vi "Oscilloscope.vi"() -> ()   [LabVIEW 2020]
uses:
  Queues4Osc.ctl
  <instrlib>/Tektronix TDS 200 1000 2000 Series/Public/Configure/Configure Trigger (Edge).vi
  <instrlib>/Tektronix TDS 200 1000 2000 Series/Tektronix TDS 200 1000 2000 Series.lvlib
panel:
  in  "VISA resource name":refnum<visa-resource-name>
  in  "stop":bool
  in  "Auto Set":bool
  in  "Measure Parameters":T1 {"Measurement Type" items=["Frequency"=0, "Period"=2, "Pk-Pk"=4, "Cycle RMS"=5]}
  in  "Trigger Parameters":T2 {"Trigger Level" min=-200.0 max=200.0 scale=-200.0..200.0}
  in  "Horizontal Parameters":T3 {"Horizontal Scale" items=["5ns"=200000000.0, "10ns"=100000000.0, "25ns"=40000000.0, "50ns"=20000000.0, "100ns"=10000000.0, "250ns"=4000000.0, "500ns"=2000000.0, "1us"=1e-06, "2.5us"=3e-06, "5us"=5e-06, "10us"=1e-05, "25us"=2.5e-05, "50us"=5e-05, "100us"=0.0001, "250us"=0.00025, "500us"=0.0005, "1ms"=0.001, "2.5ms"=0.0025, "5ms"=0.005, "10ms"=0.01, "25ms"=0.025, "50ms"=0.05, "100ms"=0.1, "250ms"=0.25, "500ms"=0.5, "1s"=1.0, "2.5s"=2.5, "5s"=5.0, "10s"=10.0, "25s"=25.0, "50s"=50.0]; "Horizontal Position" min=-1.0 max=1.0 scale=-1.0..1.0}
  in  "Vertical Parameters":T4 {"Ch2 Vertical Scale" items=["20mV"=500.0, "50mV"=200.0, "100mV"=100.0, "200mV"=50.0, "500mV"=20.0, "1V"=10.0, "2V"=5.0, "5V"=2.0, "10V"=1.0, "20V"=0.5, "50V"=0.2]; "Ch1 Vertical Scale" items=["20mV"=500.0, "50mV"=200.0, "100mV"=100.0, "200mV"=50.0, "500mV"=20.0, "1V"=10.0, "2V"=5.0, "5V"=2.0, "10V"=1.0, "20V"=0.5, "50V"=0.2]}
  out "Channel 2":waveform(dbl)(graph)
  out "Channel 1":waveform(dbl)(graph)
  # "Measure Parameters"
  # "Trigger Parameters"
  # "Horizontal Parameters"
  # "Vertical Parameters"
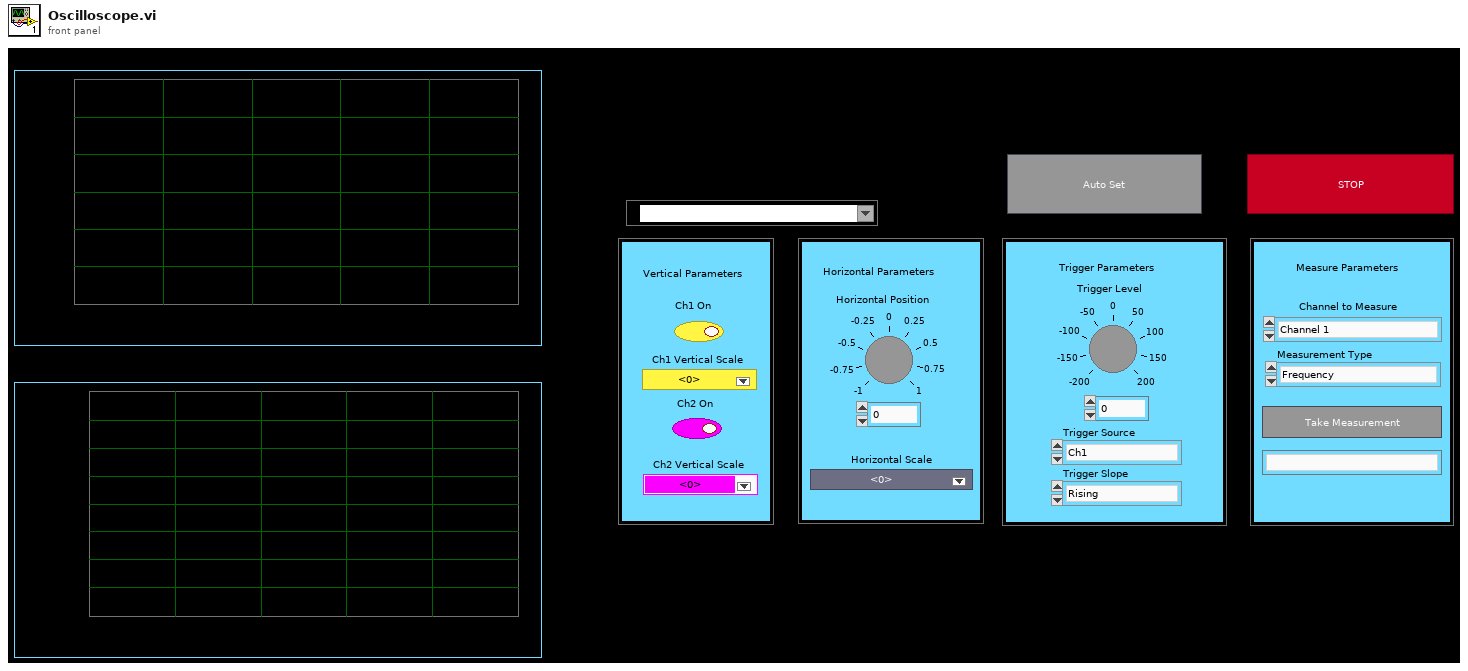
[diagram p1: front panel]
types:
  T1 = cluster{"Channel to Measure":enum16{"Channel 1", "Channel 2"}, "Take Measurement":bool, "String":string, "Measurement Type":u16}
  T2 = cluster{"Trigger Level":dbl, "Trigger Source":enum16{"Ch1", "Ch2"}, "Trigger Slope":enum16{"Rising", "Falling"}}
  T3 = cluster{"Horizontal Position":dbl, "Horizontal Scale":dbl}
  T4 = cluster{"Ch1 On":bool, "Ch2 On":bool, "Ch1 Vertical Scale":dbl, "Ch2 Vertical Scale":dbl}
  T5 = typedef "Queues4Osc.ctl" = enum16{"Initialize", "Idle", "Channels", "Horizontal", "Trigger", "Measure", "Autoset", "Stop"}
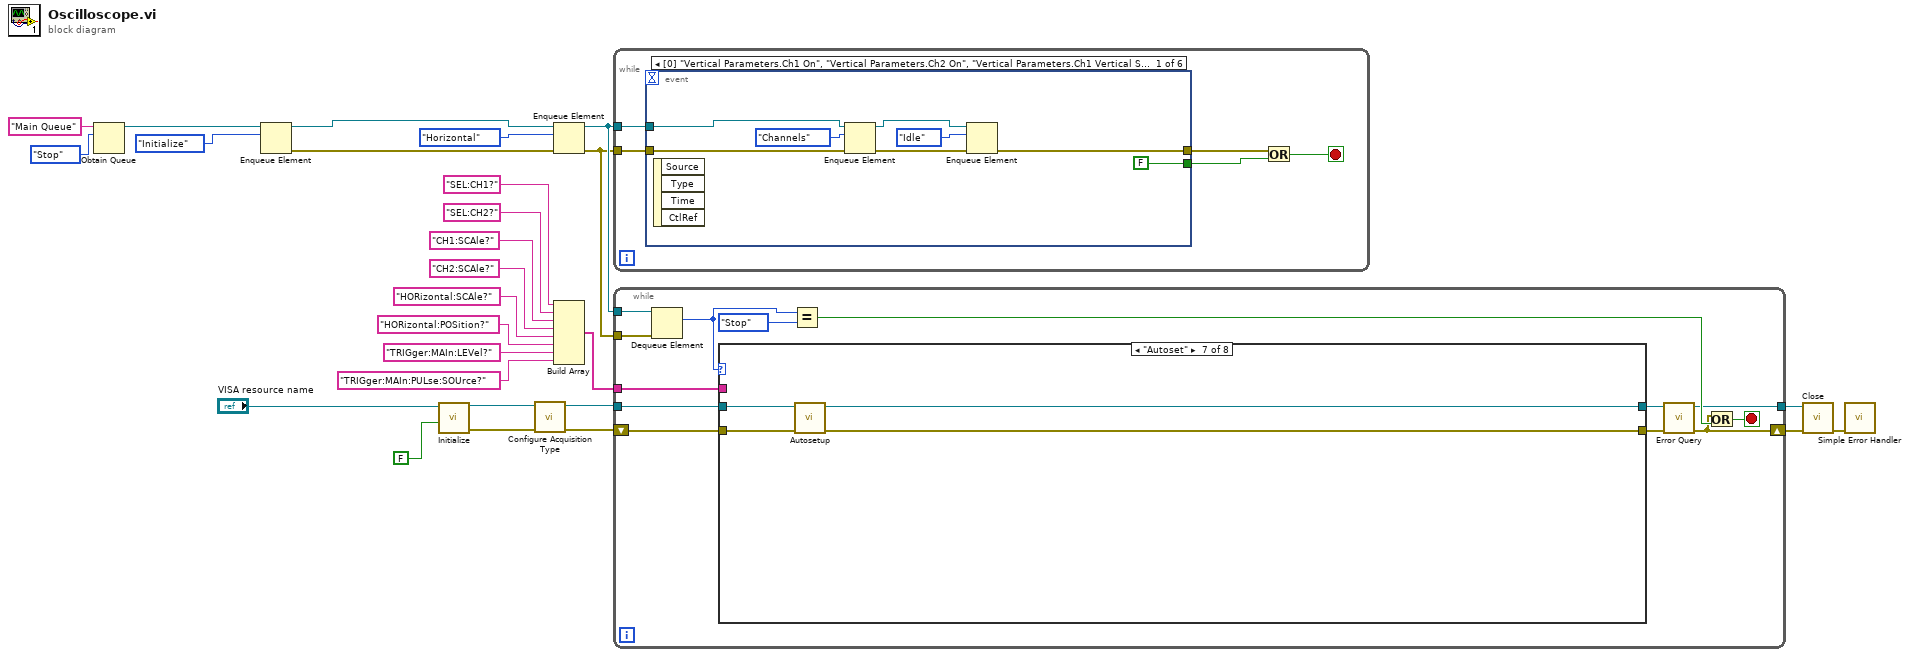
[diagram p0: block diagram]
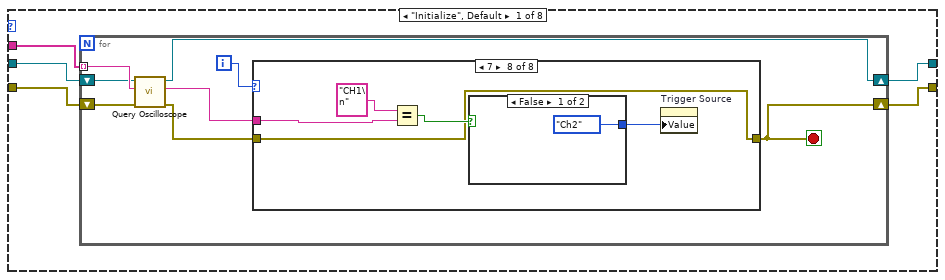
[diagram p2: hidden frame]
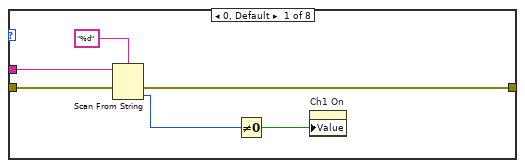
[diagram p3: hidden frame]
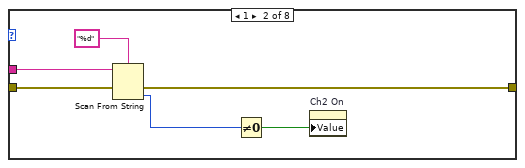
[diagram p4: hidden frame]
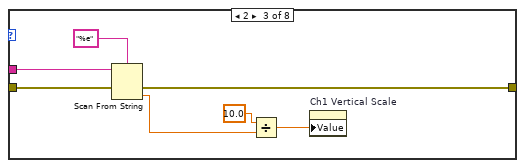
[diagram p5: hidden frame]
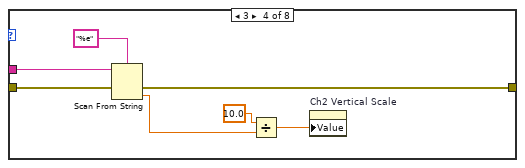
[diagram p6: hidden frame]
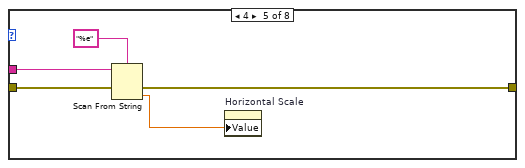
[diagram p7: hidden frame]
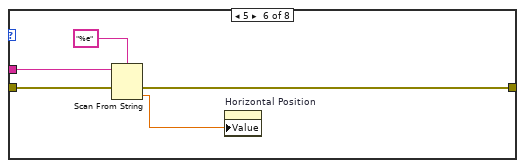
[diagram p8: hidden frame]
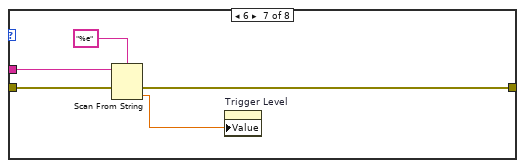
[diagram p9: hidden frame]
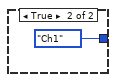
[diagram p10: hidden frame]
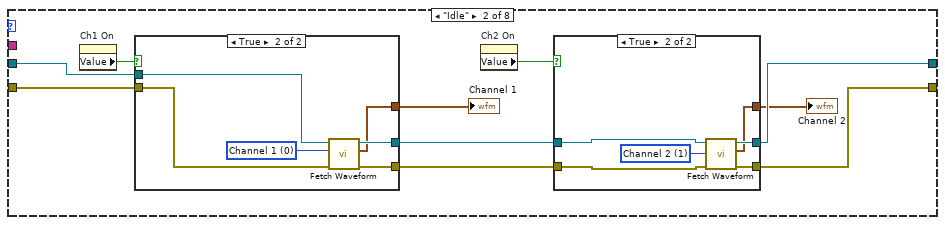
[diagram p11: hidden frame]
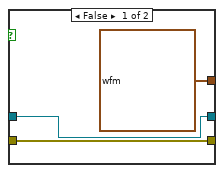
[diagram p12: hidden frame]
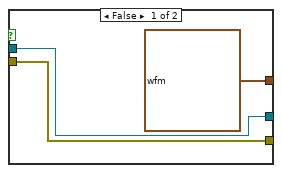
[diagram p13: hidden frame]
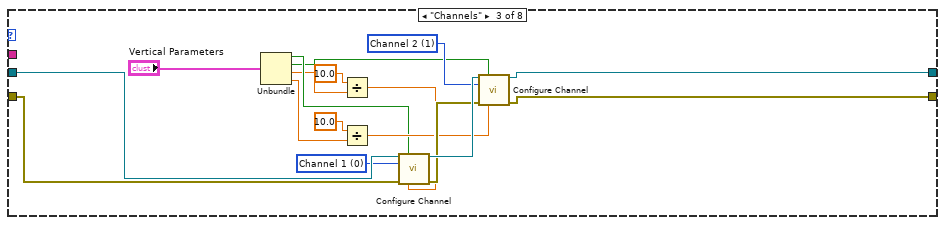
[diagram p14: hidden frame]
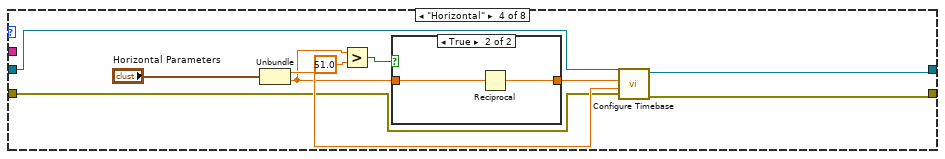
[diagram p15: hidden frame]
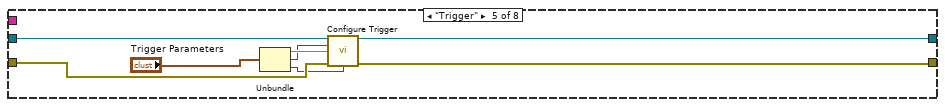
[diagram p17: hidden frame]
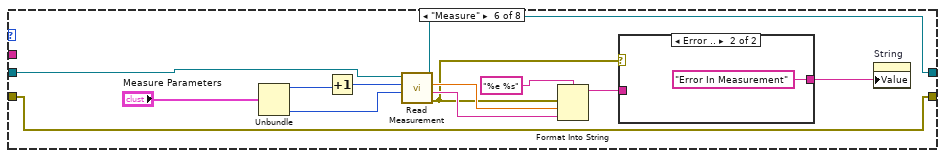
[diagram p18: hidden frame]
diagram:
  n1 = Obtain Queue(name (unnamed)="Main Queue", element data type=Queues4Osc."Stop") -> (queue out=w25:refnum<queue>)  [unwired: 3 in, 2 out]
  n2 = Enqueue Element(queue=w25, element=Queues4Osc."Initialize") -> (queue out=w8:refnum<queue>, error out=w9:errorcluster)  [unwired: 2 in, 1 out]
  n3 = call <instrlib>:"Initialize.vi"("Reset? (T: Yes)"=FALSE, "VISA resource name"="VISA resource name") -> ("error out"=w1:errorcluster, "VISA resource name out"=w2:refnum<visa-resource-name>)  [unwired: 8 in]
  n4 = call <instrlib>:"Configure Acquisition Type.vi"("error in (no error)"=w1, "VISA resource name"=w2) -> ("error out"=w3:errorcluster, "VISA resource name out"=w4:refnum<visa-resource-name>)  [unwired: 8 in]
  n5 = Enqueue Element(queue=w8, element=Queues4Osc."Horizontal", error in (no error)=w9) -> (queue out=w6:refnum<queue>, error out=w5:errorcluster)  [unwired: 1 in, 1 out]
  n6 = Build Array("SEL:CH1?" ("Input Command"), "SEL:CH2?", "CH1:SCAle?", "CH2:SCAle?", "HORizontal:SCAle?", "HORizontal:POSition?", "TRIGger:MAIn:LEVel?", "TRIGger:MAIn:PULse:SOUrce?") -> (w11:string[])
  n7 = while {
    tunnel: w6 -> [w32]
    tunnel: w5 -> [w31]
    stop <- w30 stop-if-true
    n8 = event shown="[0] \"Vertical Parameters.Ch1 On\", \"Vertical Parameters.Ch2 On\", \"Vertical Parameters.Ch1 Vertical Scale\", \"Vertical Parameters.Ch2 Vertical Scale\": Value Change" {
      selector: _ -> [_ _ _ _ _ _]
      dyn-events: _ -> [_ _ _ _ _ _]
      timeout: _ -> [_ _ _ _ _ _]
      tunnel: w32 -> [w40 w44 w52 w60 w71 w79]
      tunnel: w31 -> [w39 w43 w51 w59 w70 w78]
      tunnel: [FALSE FALSE FALSE FALSE FALSE TRUE] -> w29
      tunnel: [w33 w42 w50 w58 w65 w77] -> w28
      event "Vertical Parameters.Ch1 On", "Vertical Parameters.Ch2 On", "Vertical Parameters.Ch1 Vertical Scale", "Vertical Parameters.Ch2 Vertical Scale": Value Change {
        n9 = event-data() -> ()  [unwired: 1 in, 4 out]
        n10 = Enqueue Element(queue=w40, element=Queues4Osc."Channels", error in (no error)=w39) -> (queue out=w37:refnum<queue>, error out=w36:errorcluster)  [unwired: 1 in, 1 out]
        n11 = Enqueue Element(queue=w37, element=Queues4Osc."Idle", error in (no error)=w36) -> (error out=w33:errorcluster)  [unwired: 1 in, 2 out]
      }
      event "Horizontal Parameters.Horizontal Position", "Horizontal Parameters.Horizontal Scale": Value Change {
        n12 = event-data() -> ()  [unwired: 1 in, 4 out]
        n13 = Enqueue Element(queue=w44, element=Queues4Osc."Horizontal", error in (no error)=w43) -> (queue out=w47:refnum<queue>, error out=w48:errorcluster)  [unwired: 1 in, 1 out]
        n14 = Enqueue Element(queue=w47, element=Queues4Osc."Idle", error in (no error)=w48) -> (error out=w42:errorcluster)  [unwired: 1 in, 2 out]
      }
      event "Trigger Parameters.Trigger Level", "Trigger Parameters.Trigger Source", "Trigger Parameters.Trigger Slope": Value Change {
        n15 = event-data() -> ()  [unwired: 1 in, 4 out]
        n16 = Enqueue Element(queue=w52, element=Queues4Osc."Trigger", error in (no error)=w51) -> (queue out=w55:refnum<queue>, error out=w56:errorcluster)  [unwired: 1 in, 1 out]
        n17 = Enqueue Element(queue=w55, element=Queues4Osc."Idle", error in (no error)=w56) -> (error out=w50:errorcluster)  [unwired: 1 in, 2 out]
      }
      event "Measure Parameters.Take Measurement": Value Change {
        n18 = event-data() -> ()  [unwired: 1 in, 4 out]
        n19 = Enqueue Element(queue=w60, element=Queues4Osc."Measure", error in (no error)=w59) -> (queue out=w63:refnum<queue>, error out=w64:errorcluster)  [unwired: 1 in, 1 out]
        n20 = Enqueue Element(queue=w63, element=Queues4Osc."Idle", error in (no error)=w64) -> (error out=w58:errorcluster)  [unwired: 1 in, 2 out]
      }
      event "Auto Set": Value Change {
        n21 = event-data() -> ()  [unwired: 1 in, 4 out]
        n22 = Enqueue Element(queue=w71, element=Queues4Osc."Autoset", error in (no error)=w70) -> (queue out=w74:refnum<queue>, error out=w75:errorcluster)  [unwired: 1 in, 1 out]
        n23 = Enqueue Element(queue=w74, element=Queues4Osc."Initialize", error in (no error)=w75) -> (queue out=w68:refnum<queue>, error out=w67:errorcluster)  [unwired: 1 in, 1 out]
        n24 = Enqueue Element(queue=w68, element=Queues4Osc."Idle", error in (no error)=w67) -> (error out=w65:errorcluster)  [unwired: 1 in, 2 out]
      }
      event "stop": Value Change {
        n25 = event-data() -> ()  [unwired: 1 in, 4 out]
        n26 = Enqueue Element(queue=w79, element=Queues4Osc."Stop", error in (no error)=w78) -> (error out=w77:errorcluster)  [unwired: 1 in, 2 out]
      }
    }
    n27 = Or(x=w28, y=w29) -> (x .or. y?=w30:bool)
  }
  n28 = while {
    tunnel: w6 -> [w93]
    tunnel: w5 -> [w92]
    tunnel: [w87] -> w22
    tunnel: w4 -> [w83]
    tunnel: w11 -> [w81]
    shift-right: [w86] -> w21
    shift-left: w3 -> [w82]
    stop <- w88 stop-if-true
    n29 = Dequeue Element(queue=w93, error in (no error)=w92) -> (element=w90:T5)  [unwired: 1 in, 3 out]
    n30 = case shown="\"Autoset\"" w90 {
      tunnel: [w95 w161 w197 w203 w218 w229 w237 w241] -> w85
      tunnel: [w94 w160 w196 w202 w217 w225 w236 w240] -> w84
      tunnel: w83 -> [w97 w156 w195 w201 w220 w230 w239 w241]
      tunnel: w82 -> [w96 w155 w194 w200 w219 w225 w238 w240]
      tunnel: w81 -> [w98 _ _ _ _ _ _ _]
      frame "Initialize", Default {
        n31 = for {
          tunnel: w98 -> [w106] mode=indexing
          shift-right: [w103] -> w95
          shift-left: w97 -> [w105]
          shift-right: [w99] -> w94
          shift-left: w96 -> [w104]
          i -> [w102]
          stop <- w99 stop-if-true
          n32 = call "Query Oscilloscope.vi"("error in (no error)"=w104, "Input Command"=w106, "VISA resource name"=w105) -> ("error out"=w100:errorcluster, "read buffer"=w101:string, "VISA resource out"=w103:refnum<visa-resource-name>)  [unwired: 5 in]
          n33 = case shown="7" w102 {
            tunnel: w101 -> [w112 w115 w123 w131 w136 w140 w145 w152]
            tunnel: w100 -> [w108 w116 w124 w130 w134 w139 w146 w149]
            tunnel: [w107 w114 w122 w129 w135 w141 w144 w149] -> w99
            frame 0, Default {
              n34 = Scan From String(format string="%d", input string=w112, error in=w108) -> (error out=w107:errorcluster, output 1=w109:i32)  [unwired: 2 in, 2 out]
              n35 = Not Equal To 0?(x=w109) -> (x != 0?=w110:bool)
              n36 = property on="Ch1 On" class="Bool (strict)"("Value"=w110) -> ()  [unwired: 2 in, 2 out]
            }
            frame 1 {
              n37 = Scan From String(format string="%d", input string=w115, error in=w116) -> (error out=w114:errorcluster, output 1=w118:i32)  [unwired: 2 in, 2 out]
              n38 = Not Equal To 0?(x=w118) -> (x != 0?=w113:bool)
              n39 = property on="Ch2 On" class="Bool (strict)"("Value"=w113) -> ()  [unwired: 2 in, 2 out]
            }
            frame 2 {
              n40 = Scan From String(format string="%e", input string=w123, error in=w124) -> (error out=w122:errorcluster, output 1=w121:dbl)  [unwired: 2 in, 2 out]
              n41 = Divide(x=10.0, y=w121) -> (x/y=w119:dbl)
              n42 = property on="Ch1 Vertical Scale" class="Ring (strict)"("Value"=w119) -> ()  [unwired: 2 in, 2 out]
            }
            frame 3 {
              n43 = Scan From String(format string="%e", input string=w131, error in=w130) -> (error out=w129:errorcluster, output 1=w128:dbl)  [unwired: 2 in, 2 out]
              n44 = Divide(x=10.0, y=w128) -> (x/y=w127:dbl)
              n45 = property on="Ch2 Vertical Scale" class="Ring (strict)"("Value"=w127) -> ()  [unwired: 2 in, 2 out]
            }
            frame 4 {
              n46 = Scan From String(format string="%e", input string=w136, error in=w134) -> (error out=w135:errorcluster, output 1=w133:dbl)  [unwired: 2 in, 2 out]
              n47 = property on="Horizontal Scale" class="Ring (strict)"("Value"=w133) -> ()  [unwired: 2 in, 2 out]
            }
            frame 5 {
              n48 = Scan From String(format string="%e", input string=w140, error in=w139) -> (error out=w141:errorcluster, output 1=w138:dbl)  [unwired: 2 in, 2 out]
              n49 = property on="Horizontal Position" class="Knob (strict)"("Value"=w138) -> ()  [unwired: 2 in, 2 out]
            }
            frame 6 {
              n50 = Scan From String(format string="%e", input string=w145, error in=w146) -> (error out=w144:errorcluster, output 1=w143:dbl)  [unwired: 2 in, 2 out]
              n51 = property on="Trigger Level" class="Knob (strict)"("Value"=w143) -> ()  [unwired: 2 in, 2 out]
            }
            frame 7 {
              n52 = Equal?(x="CH1\n", y=w152) -> (x = y?=w150:bool)
              n53 = case shown="False" w150 {
                tunnel: [enum16{"Ch1", "Ch2"}."Ch2" ("Value") enum16{"Ch1", "Ch2"}."Ch1" ("Value")] -> w148
                frame False {
                }
                frame True {
                }
              }
              n54 = property on="Trigger Source" class="Enum (strict)"("Value"=w148) -> ()  [unwired: 2 in, 2 out]
            }
          }
        }
      }
      frame "Idle" {
        n55 = property on="Ch1 On" class="Bool (strict)"() -> ("Value"=w164:bool)  [unwired: 2 in, 2 out]
        n56 = case shown="True" w164 {
          tunnel: w156 -> [w176 w182]
          tunnel: w155 -> [w175 w181]
          tunnel: [w176 w179] -> w163
          tunnel: [w175 w178] -> w162
          tunnel: [waveform(dbl) {"t0"=timestamp(0 s since 1904-01-01), "dt"=1.0, "Y"=[]} ("Waveform Data") w177] -> w157
          frame False {
          }
          frame True {
            w180 = 0 items=["Channel 1", "Channel 2", "Channel 3", "Channel 4", "Math", "Reference A", "Reference B", "Reference C", "Reference D", "FFT"] ("Source (0: Channel 1)")
            n57 = call <instrlib>:"Fetch Waveform.vi"("error in (no error)"=w181, "Source (0: Channel 1)"=w180, "VISA resource name"=w182) -> ("error out"=w178:errorcluster, "Waveform Data"=w177:waveform(dbl), "VISA resource name out"=w179:refnum<visa-resource-name>)  [unwired: 6 in]
          }
        }
        "Channel 1" <- w157
        n58 = property on="Ch2 On" class="Bool (strict)"() -> ("Value"=w159:bool)  [unwired: 2 in, 2 out]
        n59 = case shown="True" w159 {
          tunnel: w163 -> [w167 w173]
          tunnel: w162 -> [w166 w172]
          tunnel: [w167 w171] -> w161
          tunnel: [w166 w170] -> w160
          tunnel: [waveform(dbl) {"t0"=timestamp(0 s since 1904-01-01), "dt"=1.0, "Y"=[]} ("Waveform Data") w169] -> w158
          frame False {
          }
          frame True {
            w168 = 1 items=["Channel 1", "Channel 2", "Channel 3", "Channel 4", "Math", "Reference A", "Reference B", "Reference C", "Reference D", "FFT"] ("Source (0: Channel 1)")
            n60 = call <instrlib>:"Fetch Waveform.vi"("error in (no error)"=w172, "Source (0: Channel 1)"=w168, "VISA resource name"=w173) -> ("error out"=w170:errorcluster, "Waveform Data"=w169:waveform(dbl), "VISA resource name out"=w171:refnum<visa-resource-name>)  [unwired: 6 in]
          }
        }
        "Channel 2" <- w158
      }
      frame "Channels" {
        w192 = 1 items=["Channel 1", "Channel 2", "Channel 3", "Channel 4", "Math", "Reference A", "Reference B", "Reference C", "Reference D"] ("Channel (0: Channel 1)")
        w193 = 0 items=["Channel 1", "Channel 2", "Channel 3", "Channel 4", "Math", "Reference A", "Reference B", "Reference C", "Reference D"] ("Channel (0: Channel 1)")
        n61 = Unbundle("Vertical Parameters") -> ("Ch1 On"=w187:bool, "Ch2 On"=w186:bool, "Ch1 Vertical Scale"=w185:dbl, "Ch2 Vertical Scale"=w184:dbl)
        n62 = Divide(x=10.0, y=w185) -> (x/y=w191:dbl)
        n63 = Divide(x=10.0, y=w184) -> (x/y=w189:dbl)
        n64 = call <instrlib>:"Configure Channel.vi"("VISA resource name"=w195, "Enable Channel (True)"=w187, "Channel (0: Channel 1)"=w193, "error in (no error)"=w194, "Vertical Range (10.0 V/div)"=w191) -> ("VISA resource name out"=w199:refnum<visa-resource-name>, "error out"=w198:errorcluster)  [unwired: 9 in]
        n65 = call <instrlib>:"Configure Channel.vi"("VISA resource name"=w199, "Enable Channel (True)"=w186, "Channel (0: Channel 1)"=w192, "error in (no error)"=w198, "Vertical Range (10.0 V/div)"=w189) -> ("VISA resource name out"=w197:refnum<visa-resource-name>, "error out"=w196:errorcluster)  [unwired: 9 in]
      }
      frame "Horizontal" {
        n66 = Unbundle("Horizontal Parameters") -> ("Horizontal Position"=w206:dbl, "Horizontal Scale"=w205:dbl)
        n67 = Greater?(x=w205, y=51.0) -> (0:w208:bool)
        n68 = case shown="True" w208 {
          tunnel: w205 -> [w210 w212]
          tunnel: [w210 w211] -> w207
          frame False {
          }
          frame True {
            n69 = Reciprocal(x=w212) -> (1/x=w211:dbl)
          }
        }
        n70 = call <instrlib>:"Configure Timebase.vi"("error in (no error)"=w200, "Position (0.0 s)"=w206, "Timebase (0.0005 s)"=w207, "VISA resource name"=w201) -> ("error out"=w202:errorcluster, "VISA resource name out"=w203:refnum<visa-resource-name>)  [unwired: 6 in]
      }
      frame "Trigger" {
        n71 = Unbundle("Trigger Parameters") -> ("Trigger Level"=w216:dbl, "Trigger Source"=w215:enum16{"Ch1", "Ch2"}, "Trigger Slope"=w214:enum16{"Rising", "Falling"})
        n72 = call-poly <instrlib>:"Configure Trigger.vi"("VISA resource name"=w220, "Trigger Source (0: Channel 1)"=w215, "Trigger Level (0.0 V)"=w216, "error in (no error)"=w219, "Trigger Slope (0: Rising)"=w214) -> ("VISA resource name out"=w218:refnum<visa-resource-name>, "error out"=w217:errorcluster)  [unwired: 9 in]
      }
      frame "Measure" {
        n73 = Unbundle("Measure Parameters") -> ("Channel to Measure"=w228:enum16{"Channel 1", "Channel 2"}, "Measurement Type"=w221:u16)  [unwired: 2 out]
        n74 = Increment(x=w228) -> (x+1=w226:enum16{"Channel 1", "Channel 2"})
        n75 = call <instrlib>:"Read Measurement.vi"("Measurement Type (0: Frequency)"=w221, "Channel (1: Channel 1)"=w226, "VISA resource name"=w230) -> ("error out"=w224:errorcluster, "Units"=w232:string, "Measurement"=w233:dbl, "VISA resource name out"=w229:refnum<visa-resource-name>)  [unwired: 5 in]
        n76 = Format Into String(format string="%e %s", error in=w224, w233, w232) -> (resulting string=w223:string)  [unwired: 1 in, 1 out]
        n77 = case shown="Error .." w224 {
          tunnel: w223 -> [w234 _]
          tunnel: [w234 "Error In Measurement"] -> w222
          frame No Error {
          }
          frame Error {
          }
        }
        n78 = property on="String" class="Str"("Value"=w222) -> ()  [unwired: 2 in, 2 out]
      }
      frame "Autoset" {
        n79 = call <instrlib>:"Autosetup.vi"("error in (no error)"=w238, "VISA resource name"=w239) -> ("error out"=w236:errorcluster, "VISA resource name out"=w237:refnum<visa-resource-name>)  [unwired: 8 in]
      }
      frame "Stop" {
      }
    }
    n80 = Equal?(x=w90, y=Queues4Osc."Stop") -> (x = y?=w89:bool)
    n81 = call <instrlib>:"Error Query.vi"("error in (no error)"=w84, "VISA resource name"=w85) -> ("error out"=w86:errorcluster, "VISA resource name out"=w87:refnum<visa-resource-name>)  [unwired: 8 out]
    n82 = Or(x=w86, y=w89) -> (x .or. y?=w88:bool)
  }
  n83 = call <instrlib>:"Close.vi"("error in (no error)"=w21, "VISA resource name"=w22) -> ("error out"=w20:errorcluster)  [unwired: 9 out]
  n84 = call <vilib>:"Simple Error Handler.vi"("error in (no error)"=w20) -> ()  [unwired: 1 in, 8 out]
